vi "CSM with INI Config.vi"(5 "Init State(\"Macro: Initialize\")":string="Macro: Initialize", 7 "Name(\"\" to use uuid)":string="CSM-Module") -> ()   [LabVIEW 2017]
uses:
  269ea9ca-c704-454f-89fe-23bfb434a412.vi
  2c2747d1-7136-4018-a18b-7ed7b9b9eea8.vi
  <userlib>/_NEVSTOP/Communicable State Machine(CSM)/AdvanceAPI/CSM - Revert Arguments-Safe String.vi
  <userlib>/_NEVSTOP/Communicable State Machine(CSM)/AdvanceAPI/CSM - Make String Arguments Safe.vi
  <userlib>/_NEVSTOP/Communicable State Machine(CSM)/AdvanceAPI/CSM - Break Down Multiple States String.vi
  <userlib>/_NEVSTOP/Communicable State Machine(CSM)/AdvanceAPI/CSM - Compact Multiple States.vi
  269ea9ca-c704-454f-89fe-23bfb434a412.vi/b09b9099-6be0-413b-8afc-4908471460c3.vi
  2c2747d1-7136-4018-a18b-7ed7b9b9eea8.vi/99de0c97-112a-4c86-9094-c187659127e1.vi
  <userlib>/_NEVSTOP/Communicable State Machine(CSM)/AdvanceAPI/CSM - Keywords.vi
  <userlib>/_NEVSTOP/Communicable State Machine(CSM)/_Shared/Trim Single-line Text.vi
  INI-Static-Variable-Support/_Support/global-csm-ini-db-change-flag.vi
  <vilib>/Utility/Data Type/Get Type Information.vi
  <userlib>/_NEVSTOP/Communicable State Machine(CSM)/addons/API-String-Arugments-Support/_Support/Data To SingleElementsArray_csm.vi
  INI-Static-Variable-Support/_Support/Parse Used Session and Name.vi
  <userlib>/_NEVSTOP/Communicable State Machine(CSM)/addons/API-String-Arugments-Support/_Support/Data To API String Arguments.vi
  INI-Static-Variable-Support/_Support/INI-FGV(lvlibp).vi
  INI-Static-Variable-Support/_Support/Populate String with INI Variable.vi
  <userlib>/_NEVSTOP/Communicable State Machine(CSM)/addons/API-String-Arugments-Support/_Support/Convert API String Arguments to Data(variant).vi
  <userlib>/_NEVSTOP/Communicable State Machine(CSM)/addons/API-String-Arugments-Support/_Support/SingleElementsArray To Data_csm.vi
  <userlib>/_NEVSTOP/Communicable State Machine(CSM)/Communicable State Machine.lvlib
  INI-Static-Variable-Support/INI-Static-Variable-Support.lvlib
panel:
  in  "string":string
  out "State History":string
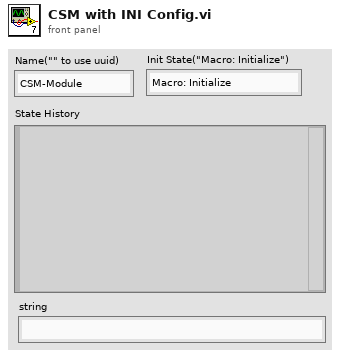
[diagram p1: front panel]
types:
  T1 = enum32{"Invalid", "Standard", "Closed", "Hidden", "Minimized", "Maximized"}
  T2 = enum32{"invalid app kind", "Development System", "Run Time System", "Student Edition", "Embedded LabVIEW", "Evaluation", "Custom"}
  T3 = typedef "Communicable State Machine.lvlib/_CSM_Response Source Message.ctl" = cluster{"‘State":string, "’Arguments":string, "’Error":errorcluster}
  T4 = cluster{"Core":cluster{"Current VI Reference":refnum<vi>, "Close Panel on Exit?":bool}, "Address":cluster{"IP":string, "Port":i16}, "Cert":cluster{"User":string, "Password":string}, "xxx":string}
  T5 = cluster{"Current VI Reference":refnum<vi>, "Close Panel on Exit?":bool}
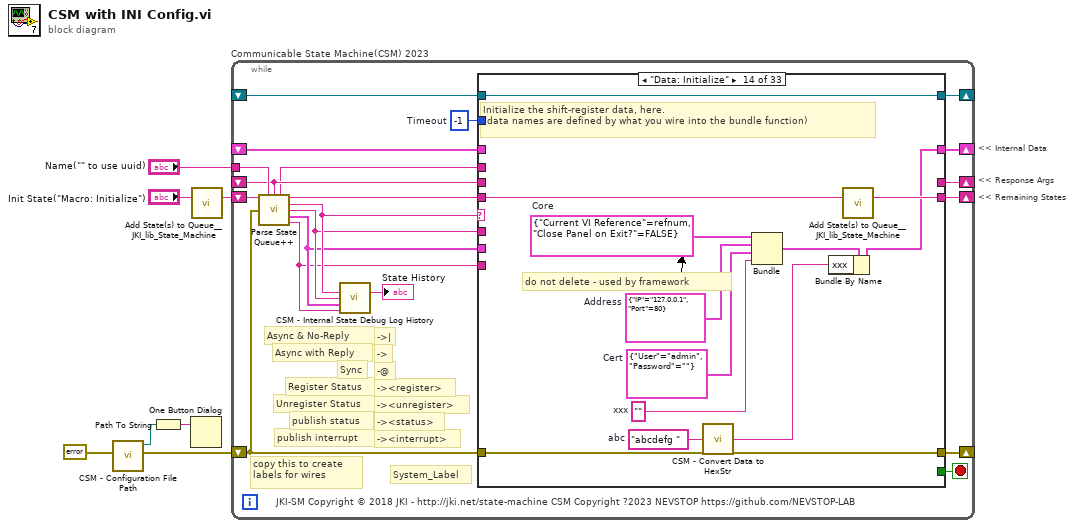
[diagram p0: block diagram]
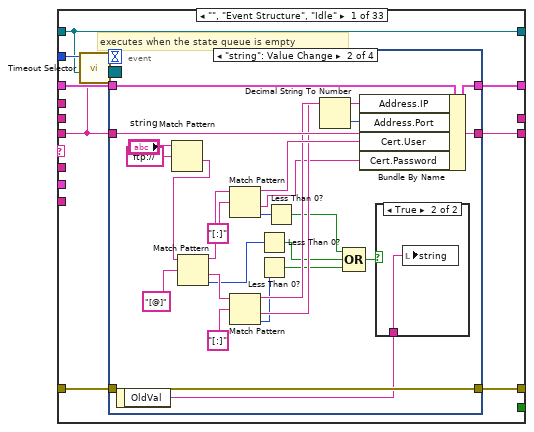
[diagram p2: hidden frame]
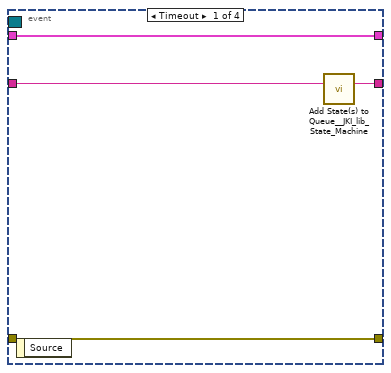
[diagram p3: hidden frame]
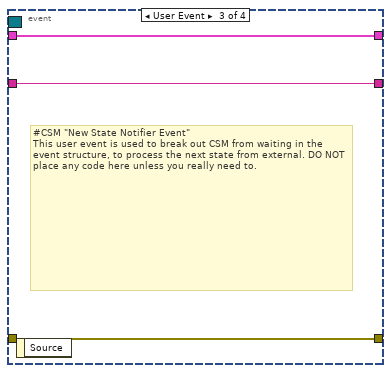
[diagram p5: hidden frame]
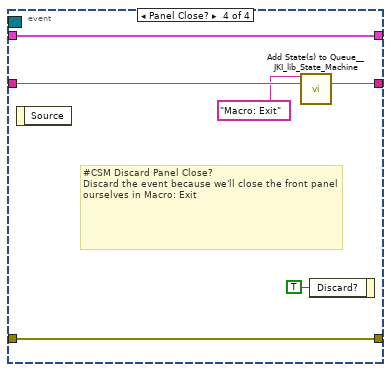
[diagram p6: hidden frame]
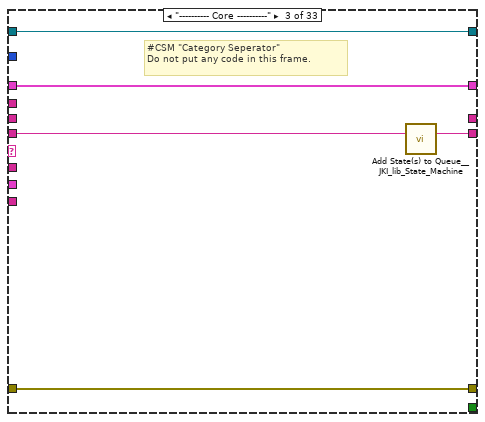
[diagram p8: hidden frame]
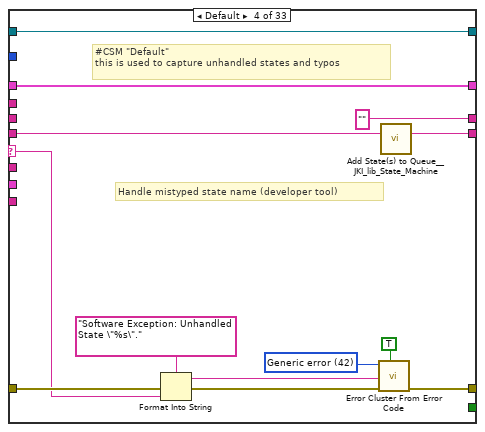
[diagram p9: hidden frame]
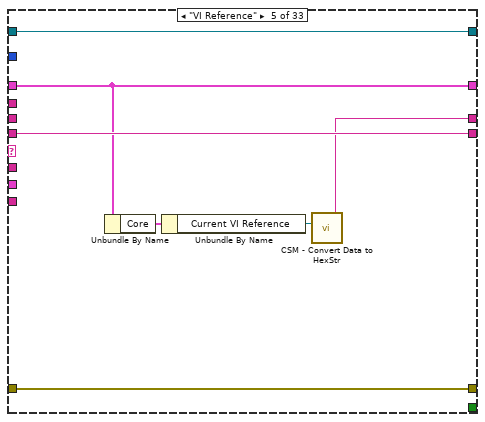
[diagram p10: hidden frame]
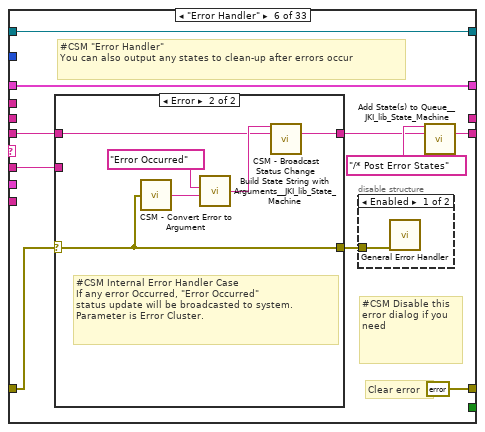
[diagram p11: hidden frame]
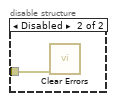
[diagram p12: hidden frame]
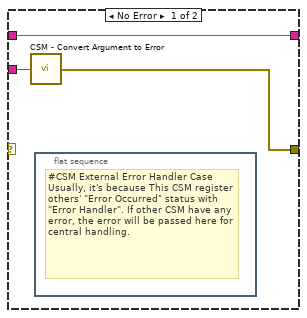
[diagram p13: hidden frame]
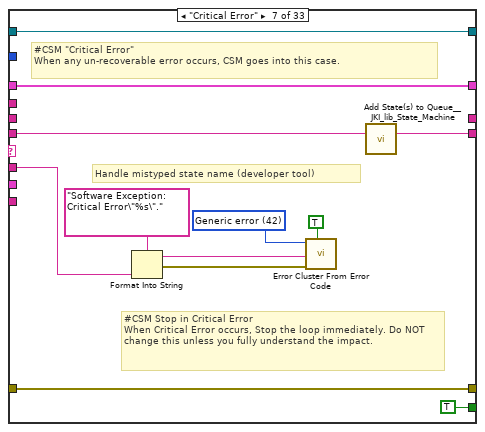
[diagram p14: hidden frame]
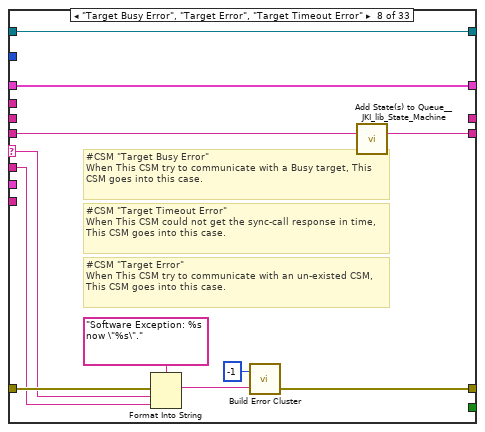
[diagram p15: hidden frame]
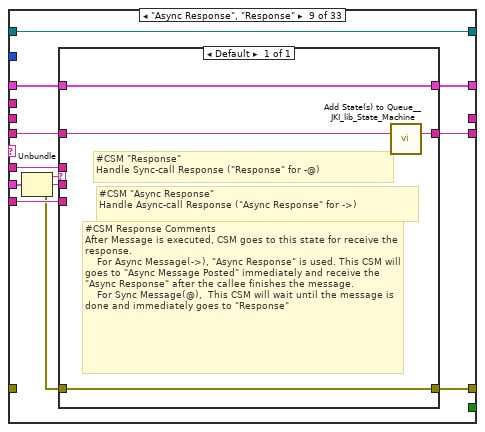
[diagram p16: hidden frame]
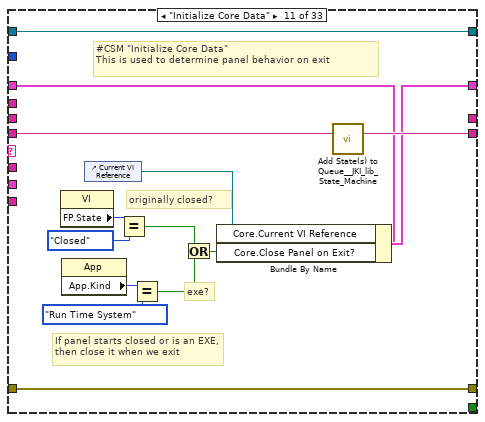
[diagram p18: hidden frame]
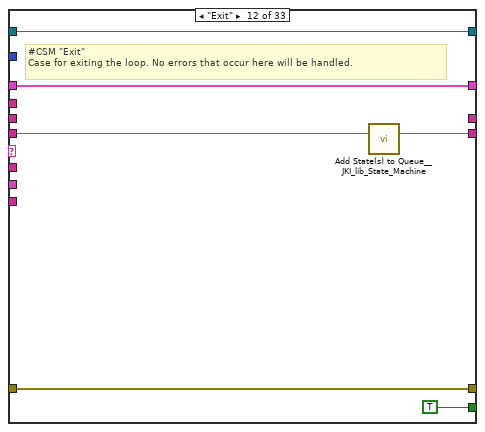
[diagram p19: hidden frame]
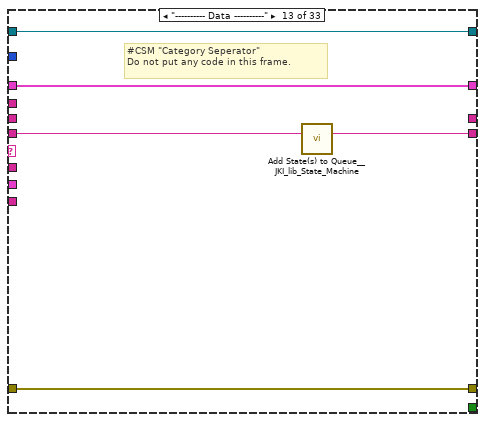
[diagram p20: hidden frame]
diagram:
  # "<< Internal Data"
  # "<< Response Args"
  # "<< Remaining States"
  n1 = call "CSM - Configuration File Path.vi"("error in (no error)"=errorcluster {"status"=FALSE, "code"=0, "source"=""} ("error out")) -> ("error out"=w3:errorcluster, "Default Config File Path"=w1:path)  [unwired: 6 in, 1 out]
  n2 = Path To String(path=w1) -> (string=w2:string)
  n3 = One Button Dialog(message=w2) -> ()  [unwired: 1 in, 1 out]
  n4 = call <vilib>:"Add State(s) to Queue__JKI_lib_State_Machine.vi"("State(s) in (\"\")"="Init State(\"Macro: Initialize\")") -> ("States Out"=w5:string)  [unwired: 14 in]
  n5 = while "Communicable State Machine(CSM) 2023" {
    shift-right: [w22] -> _
    shift-left: _ -> [w21]
    shift-right: [w25] -> _
    shift-left: w3 -> [w19]
    shift-right: [w24] -> _
    shift-left: w5 -> [w26]
    tunnel: "Name(\"\" to use uuid)" -> [w15]
    shift-right: [w18] -> _
    shift-left: _ -> [w10]
    shift-right: [w17] -> _
    shift-left: _ -> [w16]
    stop <- w23 stop-if-true
    w20 = -1  # Timeout
    # "-><interrupt>"
    # "-><status>"
    # "-><unregister>"
    # "-><register>"
    # "-@"
    # "->"
    # "->|"
    # "publish interrupt"
    # "publish status"
    # "Unregister Status"
    # "Register Status"
    # "Sync"
    # "Async with Reply"
    # "Async & No-Reply"
    # "copy this to create labels for wires"
    # "System_Label"
    # "JKI-SM Copyright © 2018 JKI - http://jki.net/state-machine CSM Copyright ?2023 NEVSTOP https://github.com/NEVSTOP-LAB"
    n6 = call <userlib>:"Parse State Queue++.vi"("State Queue"=w26, "Name (\"\" to Use UUID)"=w15, "Response Arguments"=w10, "Previous Error"=w19) -> ("Name Used"=w9:string, "Remaining States"=w27:string, "Current State"=w14:string, "Arguments"=w13:string, ">> Response Source Message >>"=w12:T3, ">> Source CSM >>"=w11:string)  [unwired: 6 in]
    n7 = call <userlib>:"CSM - Internal State Debug Log History.vi"("State"=w14, "Arguments (\"\")"=w13, ">> Response Source Message >>"=w12, "Source (\"\")"=w11) -> ("Debug Log"=→"State History":string)  [unwired: 11 in]
    n8 = case shown="\"Data: Initialize\"" w14 {
      selector: w14 -> [_ _ _ w87 _ _ _ w141 _ _ _ _ _ _ _ _ _ _ _ _ _ _ _ _ _ _ _ _ _ _ _ _ _]
      tunnel: w27 -> [w28 w78 w84 w91 w103 w109 w135 w143 w154 w167 w182 w188 w193 w205 w210 w217 w224 w229 w236 w240 w246 w257 w264 w280 w350 w356 w368 w371 w376 w382 w390 w396 w402]
      tunnel: w13 -> [_ _ _ _ _ w108 w128 w142 w153 _ _ _ _ _ _ _ _ _ _ _ _ _ w259 w274 _ _ _ _ _ w379 _ _ _]
      tunnel: w21 -> [w35 w77 w81 w89 w102 w113 w136 w145 w156 w166 w175 w186 w190 _ w208 w212 w219 w226 w235 w239 w243 w253 w262 w276 w347 w353 w365 w370 w375 w381 w387 w393 w399]
      tunnel: [w34 w79 w82 w93 w104 errorcluster {"status"=FALSE, "code"=0, "source"=""} ("error out") w137 w139 w159 w168 w179 w185 w191 w202 w211 w215 w220 w227 w230 w238 w244 w255 w260 w277 w348 w354 w366 w372 w377 w383 w388 w394 w400] -> w25
      tunnel: w19 -> [w33 w79 w82 w92 w104 w110 w137 w147 _ w168 w179 w185 w191 w202 w211 _ w221 w227 _ w241 w244 w255 w261 w278 w348 w354 w366 w372 w377 w383 w388 w394 w400]
      tunnel: [w36 w78 w83 w90 w103 w105 w134 w146 w155 w167 w181 w187 w192 w204 w210 w217 w223 w228 w236 w240 w245 w256 w263 w279 w349 w355 w367 w371 w376 w382 w389 w395 w401] -> w24
      tunnel: [_ _ _ _ _ _ TRUE _ _ _ _ TRUE _ _ _ _ _ _ _ _ _ _ _ _ _ _ _ _ _ _ _ _ _] -> w23
      tunnel: [w32 w77 w81 w89 w102 w113 w136 w145 w157 w166 w180 w186 w190 w195 w207 w213 w219 w226 w235 w239 w243 w253 w262 w276 w347 w353 w365 w370 w375 w381 w387 w393 w399] -> w22
      tunnel: w20 -> [w31 _ _ _ _ _ _ _ _ _ _ _ _ _ _ _ _ _ _ _ _ _ _ _ _ _ _ _ _ _ _ _ _]
      tunnel: w11 -> [_ _ _ _ _ _ _ _ w151 _ _ _ _ _ _ _ _ _ _ _ _ _ _ _ _ _ _ _ _ _ _ _ _]
      tunnel: w12 -> [_ _ _ _ _ _ _ _ w158 _ _ _ _ _ _ _ _ _ _ _ _ _ _ _ _ _ _ _ _ _ _ _ _]
      tunnel: [_ _ _ "" w98 _ _ _ _ _ _ _ _ _ _ _ _ _ _ _ _ _ _ _ _ _ _ _ "API1 Response" w378 _ "DoA Finished" "DoB Finished"] -> w18
      tunnel: [w30 w76 w80 w85 w101 w112 w126 w144 w160 w165 w169 w183 w189 w200 w209 w216 w218 w225 w234 w237 w242 w254 w258 w273 w346 w351 w358 w369 w374 w380 w386 w392 w398] -> w17
      tunnel: w16 -> [w30 w76 w80 w85 w101 w112 w126 w144 w160 w165 w169 w183 w189 w200 w209 w216 w218 w225 _ w237 w242 w254 w258 w273 w346 w351 w358 w369 w374 w380 w386 w392 w398]
      tunnel: w10 -> [_ _ _ _ _ _ _ _ _ _ _ _ _ _ _ _ _ _ _ _ _ _ _ _ _ _ _ _ _ _ _ _ _]
      tunnel: w9 -> [_ _ _ _ _ _ _ _ _ _ _ _ _ _ w206 w214 _ _ w233 _ _ _ _ _ _ _ _ _ _ _ _ _ _]
      frame "", "Event Structure", "Idle" {
        # "executes when the state queue is empty"
        n9 = call <userlib>:"Timeout Selector.vi"("Remaining States"=w28, "Timeout Expected"=w31) -> ("Timeout"=w29:i32)  [unwired: 5 in]
        n10 = event shown="[1] \"string\": Value Change" {
          selector: w30 -> [_ _ _ _]
          dyn-events: _ -> [_ _ _ _]
          timeout: w29 -> [_ _ _ _]
          tunnel: w28 -> [w40 w65 w68 w75]
          tunnel: [w39 w65 w68 w74] -> w36
          tunnel: w35 -> [w37 w63 w69 w72]
          tunnel: [w38 w64 w67 w73] -> w34
          tunnel: w33 -> [w38 w64 w67 w73]
          tunnel: [w37 w61 w69 w72] -> w32
          event Timeout {
            n11 = event-data() -> ()  [unwired: 1 in, 1 out]
            n12 = call <vilib>:"Add State(s) to Queue__JKI_lib_State_Machine.vi"("State(s) in (\"\")"=w40) -> ("States Out"=w39:string)  [unwired: 14 in]
          }
          event "string": Value Change {
            n13 = event-data() -> ("OldVal"=w62:string)  [unwired: 1 in]
            n14 = Match Pattern(string="string", regular expression="ftp://") -> (after substring=w42:string)  [unwired: 1 in, 3 out]
            n15 = Match Pattern(string=w42, regular expression="[@]") -> (before substring=w58:string, after substring=w56:string, offset past match=w51:i32)  [unwired: 1 in, 1 out]
            n16 = Match Pattern(string=w58, regular expression="[:]") -> (before substring=w55:string, after substring=w41:string, offset past match=w50:i32)  [unwired: 1 in, 1 out]
            n17 = Match Pattern(string=w56, regular expression="[:]") -> (before substring=w54:string, after substring=w53:string, offset past match=w49:i32)  [unwired: 1 in, 1 out]
            n18 = Less Than 0?(x=w51) -> (x < 0?=w46:bool)
            n19 = Less Than 0?(x=w49) -> (x < 0?=w45:bool)
            n20 = Less Than 0?(x=w50) -> (x < 0?=w47:bool)
            n21 = Decimal String To Number(string=w53) -> (number=w52:i32)  [unwired: 2 in, 1 out]
            n22 = Compound Arithmetic op=OR(w47, w46, w45) -> (w48:bool)
            n23 = Bundle By Name(cluster=w63, "Address.IP"=w54, "Address.Port"=w52, "Cert.User"=w55, "Cert.Password"=w41) -> (w61:T4)
            n24 = case shown="True" w48 {
              tunnel: w62 -> [_ w66]
              frame False {
              }
              frame True {
                n25 = local write "string"(w66) -> ()
              }
            }
          }
          event User Event {
            # "#CSM \"New State Notifier Event\"\nThis user event is used to break out CSM from waiting in the event structure, to process the next state from external. DO NOT place any code here unless you really need to."
            n26 = event-data() -> ()  [unwired: 1 in, 1 out]
          }
          event Panel Close? {
            # "#CSM Discard Panel Close?\nDiscard the event because we'll close the front panel ourselves in Macro: Exit"
            n27 = event-data() -> ()  [unwired: 1 in, 1 out]
            n28 = call <vilib>:"Add State(s) to Queue__JKI_lib_State_Machine.vi"("State(s) in Front (\"\")"="Macro: Exit", "State(s) in (\"\")"=w75) -> ("States Out"=w74:string)  [unwired: 13 in]
            n29 = event-data("Discard?"=TRUE) -> ()  [unwired: 1 in, 1 out]
          }
        }
      }
      frame "CSM Documentation" {
        # "#CSM README FIRST\n\nCSM is a LabVIEW application framework that builds upon JKI State Machine (JKISM). It follows the pattern of JKISM and extends the keywords to describe message communication between CSM modules, including concepts such as Sync-Message, Async-Message, Subscription/Unsubscription of status - essential elements for creating reusable code modules. For more information, please visit the CSM wiki: https://github.com/NEVSTOP-LAB/JKI-State-Machine-Plus-Plus/wiki\n\nFor instructions on JKI State Machine, visit: http://jki.net/state-machine/\nFor information about CSM, visit: https://github.com/NEVSTOP-LAB"
        # "#CSM \"Documentation\"\nCase for holding CSM Documenation"
      }
      frame "---------- Core ----------" {
        # "#CSM \"Category Seperator\"\nDo not put any code in this frame."
        n30 = call <vilib>:"Add State(s) to Queue__JKI_lib_State_Machine.vi"("State(s) in (\"\")"=w84) -> ("States Out"=w83:string)  [unwired: 14 in]
      }
      frame Default {
        w96 = 42 items=["No error", "Argument error", "Memory is full", "Out of zone", "End of file", "File already open", "Generic file I/O error", "File not found", "File permission error", "Disk is full", "Duplicate path", "Too many files open", "System feature not enabled", "Resource file not found", "Cannot add resource", "Resource not found", "Image not found", "Image memory error", "Pen does not exist", "Config type invalid", "Config token not found", "Config parse error", "Config memory error", "Bad external code format", "Bad external code offset", "External code not present", "Null window", "Destroy window error", "Null menu", "Print aborted", "Bad print record", "Print driver error", "Windows error during printing", "Memory error during printing", "Print dialog error", "Generic print error", "Invalid device refnum", "Device not found", "Device parameter error", "Device unit error", "Cannot open device", "Device call aborted", "Generic error", "Cancelled by user", "Object ID too low", "Object ID too high", "Object not in heap", "Unknown heap", "Unknown object (invalid DefProc)", "Unknown object (DefProc not in table)", "Message out of range", "Invalid (null) method", "Unknown message", "Manager call not supported", "Bad address", "Network operation in progress", "Network operation timed out", "Connection is busy", "Network attribute not supported", "Network error", "Address in use", "System out of memory", "Connection aborted", "Connection refused", "Not connected", "Already connected", "Connection closed", "Initialization error (interapplication manager)", "Bad occurrence", "Wait on unbound occurrence handler", "Occurrence queue overflow", "Datalog type conflict", "Unused", "Unrecognized type (interapplication manager)", "Memory corrupt", "Failed to make temporary DLL", "Old CIN version", "Drag socket not found", "Failed to load drop-object", "Failed to register OLE object", "Failed to release OLE object", "Format specifier type mismatch", "Unknown format specifier", "Too few format specifiers", "Too many format specifiers", "Scan failed", "Newer CIN version", "Error converting to variant", "Runtime menu error", "Password tampered", "Variant attribute not found", "Incompatible variant data type", "Event data is not available", "Event Store is not present", "Occurrence is not found", "Event Queue is not created", "Event info is not available", "Refnum passed is NULL", "Error retrieving Class GUID", "Error retrieving CoClass GUID", "Error retrieving TypeLib GUID.", "Bad built application magic bytes.", "Specific driver is different from the specific driver associated with the Logical Name.", "There is no session opened to the class driver.", "Max Error", "MAX - Error with config objects", "MAX - Error loading configuration", "MAX - Group not supported"]
        # "#CSM \"Default\"\nthis is used to capture unhandled states and typos"
        # "Handle mistyped state name (developer tool)"
        n31 = Format Into String(format string="Software Exception: Unhandled State \"%s\"." ("message"), error in=w92, w87) -> (resulting string=w95:string, error out=w94:errorcluster)  [unwired: 1 in]
        n32 = call <vilib>:"Error Cluster From Error Code.vi"("show call chain? (False)"=TRUE, "error in (no error)"=w94, "error message (\"\")"=w95, "error code (0)"=w96) -> ("error out"=w93:errorcluster)  [unwired: 5 in]
        n33 = call <vilib>:"Add State(s) to Queue__JKI_lib_State_Machine.vi"("State(s) in (\"\")"=w91) -> ("States Out"=w90:string)  [unwired: 14 in]
      }
      frame "VI Reference" {
        n34 = Unbundle By Name(w102) -> ("Core"=w100:T5)
        n35 = Unbundle By Name(w100) -> ("Current VI Reference"=w99:refnum<vi>)
        n36 = call <userlib>:"CSM - Convert Data to HexStr.vi"("Variant"=w99) -> ("HEX String (0-9,A-F)"=w98:string)  [unwired: 8 in]
      }
      frame "Error Handler" {
        # "#CSM Disable this error dialog if you need"
        # "#CSM \"Error Handler\"\nYou can also output any states to clean-up after errors occur"
        # "Clear error"
        n37 = case shown="Error" w110 {
          selector: w110 -> [_ w120]
          tunnel: [w119 w122] -> w106
          tunnel: w109 -> [w119 w121]
          tunnel: w108 -> [w118 _]
          tunnel: [w117 w120] -> w111
          frame No Error {
            n38 = call <userlib>:"CSM - Convert Argument to Error.vi"("Argument"=w118) -> ("Error"=w117:errorcluster)  [unwired: 4 in]
            n39 = flat-sequence {
              frame #0 {
                # "#CSM External Error Handler Case\nUsually, it's because This CSM register others' \"Error Occurred\" status with \"Error Handler\". If other CSM have any error, the error will be passed here for central handling."
              }
            }
          }
          frame Error {
            # "#CSM Internal Error Handler Case \nIf any error Occurred, \"Error Occurred\" \nstatus update will be broadcasted to system.\nParameter is Error Cluster."
            n40 = call <userlib>:"CSM - Convert Error to Argument.vi"("Error"=w120) -> ("Argument"=w124:string)  [unwired: 4 in]
            n41 = call <vilib>:"Build State String with Arguments__JKI_lib_State_Machine.vi"("Arguments (\"\")"=w124, "State"="Error Occurred" ("Status with Arguments")) -> ("State with Arguments"=w123:string)  [unwired: 4 in]
            n42 = call <userlib>:"CSM - Broadcast Status Change.vi"("Status With Arguments"=w123, "State Queue"=w121) -> ("Remaining States"=w122:string)  [unwired: 13 in]
          }
        }
        n43 = disable-structure shown="Enabled" {
          disable-tunnel: w111 -> [w115 w116]
          frame Enabled {
            n44 = call <vilib>:"General Error Handler.vi"("error in (no error)"=w115) -> ()  [unwired: 10 in, 5 out]
          }
          frame Disabled {
            n45 = call <vilib>:"Clear Errors.vi"("error in (no error)"=w116) -> ()  [unwired: 5 in, 2 out]
          }
        }
        n46 = call <vilib>:"Add State(s) to Queue__JKI_lib_State_Machine.vi"("State(s) in Front (\"\")"="/* Post Error States", "State(s) in (\"\")"=w106) -> ("States Out"=w105:string)  [unwired: 13 in]
      }
      frame "Critical Error" {
        w132 = 42 items=["No error", "Argument error", "Memory is full", "Out of zone", "End of file", "File already open", "Generic file I/O error", "File not found", "File permission error", "Disk is full", "Duplicate path", "Too many files open", "System feature not enabled", "Resource file not found", "Cannot add resource", "Resource not found", "Image not found", "Image memory error", "Pen does not exist", "Config type invalid", "Config token not found", "Config parse error", "Config memory error", "Bad external code format", "Bad external code offset", "External code not present", "Null window", "Destroy window error", "Null menu", "Print aborted", "Bad print record", "Print driver error", "Windows error during printing", "Memory error during printing", "Print dialog error", "Generic print error", "Invalid device refnum", "Device not found", "Device parameter error", "Device unit error", "Cannot open device", "Device call aborted", "Generic error", "Cancelled by user", "Object ID too low", "Object ID too high", "Object not in heap", "Unknown heap", "Unknown object (invalid DefProc)", "Unknown object (DefProc not in table)", "Message out of range", "Invalid (null) method", "Unknown message", "Manager call not supported", "Bad address", "Network operation in progress", "Network operation timed out", "Connection is busy", "Network attribute not supported", "Network error", "Address in use", "System out of memory", "Connection aborted", "Connection refused", "Not connected", "Already connected", "Connection closed", "Initialization error (interapplication manager)", "Bad occurrence", "Wait on unbound occurrence handler", "Occurrence queue overflow", "Datalog type conflict", "Unused", "Unrecognized type (interapplication manager)", "Memory corrupt", "Failed to make temporary DLL", "Old CIN version", "Drag socket not found", "Failed to load drop-object", "Failed to register OLE object", "Failed to release OLE object", "Format specifier type mismatch", "Unknown format specifier", "Too few format specifiers", "Too many format specifiers", "Scan failed", "Newer CIN version", "Error converting to variant", "Runtime menu error", "Password tampered", "Variant attribute not found", "Incompatible variant data type", "Event data is not available", "Event Store is not present", "Occurrence is not found", "Event Queue is not created", "Event info is not available", "Refnum passed is NULL", "Error retrieving Class GUID", "Error retrieving CoClass GUID", "Error retrieving TypeLib GUID.", "Bad built application magic bytes.", "Specific driver is different from the specific driver associated with the Logical Name.", "There is no session opened to the class driver.", "Max Error", "MAX - Error with config objects", "MAX - Error loading configuration", "MAX - Group not supported"]
        # "#CSM Stop in Critical Error\nWhen Critical Error occurs, Stop the loop immediately. Do NOT change this unless you fully understand the impact."
        # "#CSM \"Critical Error\"\nWhen any un-recoverable error occurs, CSM goes into this case."
        # "Handle mistyped state name (developer tool)"
        n47 = Format Into String(format string="Software Exception: Critical Error\"%s\"." ("message"), w128) -> (resulting string=w131:string, error out=w130:errorcluster)  [unwired: 2 in]
        n48 = call <vilib>:"Error Cluster From Error Code.vi"("show call chain? (False)"=TRUE, "error in (no error)"=w130, "error message (\"\")"=w131, "error code (0)"=w132) -> ()  [unwired: 5 in, 1 out]
        n49 = call <vilib>:"Add State(s) to Queue__JKI_lib_State_Machine.vi"("State(s) in (\"\")"=w135) -> ("States Out"=w134:string)  [unwired: 14 in]
      }
      frame "Target Busy Error", "Target Error", "Target Timeout Error" {
        # "#CSM \"Target Error\"\nWhen This CSM try to communicate with an un-existed CSM, This CSM goes into this case."
        # "#CSM \"Target Timeout Error\"\nWhen This CSM could not get the sync-call response in time, This CSM goes into this case."
        # "#CSM \"Target Busy Error\"\nWhen This CSM try to communicate with a Busy target, This CSM goes into this case."
        n50 = Format Into String(format string="Software Exception: %s now \"%s\"." ("message"), error in=w147, w141, w142) -> (resulting string=w140:string)  [unwired: 1 in, 1 out]
        n51 = call <userlib>:"Build Error Cluster.vi"("String to Prepend to Source (\"\")"=w140, "Code"=-1 ("code")) -> ("error out"=w139:errorcluster)
        n52 = call <vilib>:"Add State(s) to Queue__JKI_lib_State_Machine.vi"("State(s) in (\"\")"=w143) -> ("States Out"=w146:string)  [unwired: 14 in]
      }
      frame "Async Response", "Response" {
        n53 = Unbundle(w158) -> ("‘State"=w152:string, "’Arguments"=w150:string, "’Error"=w149:errorcluster)
        n54 = case shown="Default" w152 {
          tunnel: [w164] -> w159
          tunnel: w149 -> [w164]
          tunnel: [w163] -> w157
          tunnel: w156 -> [w163]
          tunnel: [w161] -> w155
          tunnel: w154 -> [w162]
          tunnel: w153 -> [_]
          tunnel: w151 -> [_]
          tunnel: w150 -> [_]
          frame Default {
            # "#CSM Response Comments\nAfter Message is executed, CSM goes to this state for receive the response.\n    For Async Message(->), \"Async Response\" is used. This CSM will goes to \"Async Message Posted\" immediately and receive the \"Async Response\" after the callee finishes the message.\n    For Sync Message(@),  This CSM will wait until the message is done and immediately goes to \"Response\""
            # "#CSM \"Async Response\"\nHandle Async-call Response (\"Async Response\" for ->)"
            # "#CSM \"Response\"\nHandle Sync-call Response (\"Response\" for -@)"
            n55 = call <vilib>:"Add State(s) to Queue__JKI_lib_State_Machine.vi"("State(s) in (\"\")"=w162) -> ("States Out"=w161:string)  [unwired: 14 in]
          }
        }
      }
      frame "Async Message Posted" {
        # "#CSM \"Async Message Posted\"\nAfter Async Message is posted (-> or ->| ), CSM goes to this state for post-action.\nYou can use Argument - State to tell which Async Message is called."
      }
      frame "Initialize Core Data" {
        # "#CSM \"Initialize Core Data\"\nThis is used to determine panel behavior on exit"
        # "originally closed?"
        # "exe?"
        # "If panel starts closed or is an EXE, then close it when we exit"
        n56 = property class="VI"() -> ("FP.State"=w172:T1)  [unwired: 2 in, 2 out]
        n57 = property class="App"() -> ("App.Kind"=w178:T2)  [unwired: 2 in, 2 out]
        n58 = control-ref of="Current VI Reference"() -> (w173:refnum<vi>)
        n59 = Equal?(x=w172, y=T1."Closed" ("Front Panel Window:State")) -> (x = y?=w170:bool)
        n60 = Equal?(x=w178, y=T2."Run Time System" ("Application:Kind")) -> (x = y?=w176:bool)
        n61 = Or(x=w170, y=w176) -> (x .or. y?=w174:bool)
        n62 = Bundle By Name(cluster=w175, "Core.Current VI Reference"=w173, "Core.Close Panel on Exit?"=w174) -> (w180:T4)
        n63 = call <vilib>:"Add State(s) to Queue__JKI_lib_State_Machine.vi"("State(s) in (\"\")"=w182) -> ("States Out"=w181:string)  [unwired: 14 in]
      }
      frame "Exit" {
        # "#CSM \"Exit\"\nCase for exiting the loop. No errors that occur here will be handled."
        n64 = call <vilib>:"Add State(s) to Queue__JKI_lib_State_Machine.vi"("State(s) in (\"\")"=w188) -> ("States Out"=w187:string)  [unwired: 14 in]
      }
      frame "---------- Data ----------" {
        # "#CSM \"Category Seperator\"\nDo not put any code in this frame."
        n65 = call <vilib>:"Add State(s) to Queue__JKI_lib_State_Machine.vi"("State(s) in (\"\")"=w193) -> ("States Out"=w192:string)  [unwired: 14 in]
      }
      frame "Data: Initialize" {
        w196 = "abcdefg "  # abc
        w197 = ""  # xxx
        w198 = cluster{"User":string, "Password":string} {"User"="admin", "Password"=""}  # Cert
        w199 = cluster{"IP":string, "Port":i16} {"IP"="127.0.0.1", "Port"=80}  # Address
        w201 = T5 {"Current VI Reference"=refnum, "Close Panel on Exit?"=FALSE}  # Core
        # "do not delete - used by framework"
        # "Initialize the shift-register data, here.\n(data names are defined by what you wire into the bundle function)"
        n66 = call <userlib>:"CSM - Convert Data to HexStr.vi"("Variant"=w196) -> ("HEX String (0-9,A-F)"=w194:string)  [unwired: 8 in]
        n67 = Bundle("Core"=w201, "Address"=w199, "Cert"=w198, "xxx"=w197) -> (w203:T4)  [unwired: 1 in]
        n68 = Bundle By Name(cluster=w203, "xxx"=w194) -> (w195:T4)
        n69 = call <vilib>:"Add State(s) to Queue__JKI_lib_State_Machine.vi"("State(s) in (\"\")"=w205) -> ("States Out"=w204:string)  [unwired: 14 in]
      }
      frame "Data: Load From INI" {
        n70 = call "CSM - Read Configuration Variable.vim"("Section Name(\"\" as Default)"=w206, "config prototype(Cluster Prefered)"=w208) -> ("config out"=w207:T4)  [unwired: 6 in, 1 out]
      }
      frame "Data: Save to INI" {
        n71 = call "CSM - Write Configuration Variable.vim"("Section Name(\"\" as Default)"=w214, "Variant"=w212) -> ("error out"=w215:errorcluster, "Variant (dup)"=w213:T4)  [unwired: 6 in]
      }
      frame "Data: Cleanup" {
        # "Cleanup any data and references, here.\n(this is called automatically, by the Macro: Exit)"
        n72 = Unbundle By Name(w219) -> ("Core.Current VI Reference"=w222:refnum<vi>)
        n73 = Close Reference(reference=w222, error in (no error)=w221) -> (error out=w220:errorcluster)
        n74 = call <vilib>:"Add State(s) to Queue__JKI_lib_State_Machine.vi"("State(s) in (\"\")"=w224) -> ("States Out"=w223:string)  [unwired: 14 in]
      }
      frame "---------- Events ----------" {
        # "#CSM \"Category Seperator\"\nDo not put any code in this frame."
        n75 = call <vilib>:"Add State(s) to Queue__JKI_lib_State_Machine.vi"("State(s) in (\"\")"=w229) -> ("States Out"=w228:string)  [unwired: 14 in]
      }
      frame "Events: Register" {
        # "#CSM \"Events: Register\"\nRegister user event. New Message Event is registered to break CSM waiting in event structure by default."
        # "#CSM Register New Message Event\nRegister message event to break Waiting in Event structure."
        n76 = call <userlib>:"CSM - Get New State Notifier Event.vi"("Name (\"\" to Use UUID) In"=w233) -> ("error out"=w231:errorcluster, "New State Notifier Event"=w232:refnum<user-event>)  [unwired: 9 in]
        n77 = register-events(error in=w231, w232) -> (reference out=w234:refnum<event-registration>, error out=w230:errorcluster)  [unwired: 1 in]
      }
      frame "Events: Unregister" {
        # "#CSM \"Events: Unregister\"\nUnregister user event."
        n78 = Unregister For Events(event registration refnum=w237, error in=w241) -> (error out=w238:errorcluster)
      }
      frame "---------- UI ----------" {
        # "#CSM \"Category Seperator\"\nDo not put any code in this frame."
        n79 = call <vilib>:"Add State(s) to Queue__JKI_lib_State_Machine.vi"("State(s) in (\"\")"=w246) -> ("States Out"=w245:string)  [unwired: 14 in]
      }
      frame "UI: Initialize" {
        # "#CSM \"UI: Initialize\"\nInitialize the User Interface, here.\n(this is called automatically, by the Macro: Init)"
        n80 = Unbundle By Name(w253) -> ("Address.IP"=w249:string, "Address.Port"=w248:i16, "Cert.User"=w251:string, "Cert.Password"=w250:string)
        n81 = Format Into String(format string="ftp://%s:%s@%s:%d", w251, w250, w249, w248) -> (resulting string=w247:string)  [unwired: 2 in, 1 out]
        n82 = call <vilib>:"Add State(s) to Queue__JKI_lib_State_Machine.vi"("State(s) in (\"\")"=w257) -> ("States Out"=w256:string)  [unwired: 14 in]
        n83 = local write "string"(w247) -> ()
      }
      frame "UI: Cursor Set" {
        # "#CSM \"UI: Cursor Set\"\nSet and Unset Cursor Busy.\n(Usage: \"UI: Cursor Set >> Busy|Idle\")"
        # "Argument"
        n84 = disable-structure shown="Default" {
          disable-tunnel: w261 -> [w267 w272]
          disable-tunnel: [w266 w272] -> w260
          disable-tunnel: w259 -> [w265 _]
          frame condition #0 (active) {
            n85 = case shown="\"Idle\", Default" w265 {
              tunnel: w267 -> [w269 w271]
              tunnel: [w268 w270] -> w266
              frame "Idle", Default {
                n86 = call <vilib>:"Unset Busy.vi"("error in (no error)"=w269) -> ("error out"=w268:errorcluster)  [unwired: 10 in]
              }
              frame "Busy" {
                n87 = call <vilib>:"Set Busy.vi"("error in (no error)"=w271) -> ("error out"=w270:errorcluster)  [unwired: 9 in, 1 out]
              }
            }
          }
          frame condition #1 {
          }
        }
        n88 = call <vilib>:"Add State(s) to Queue__JKI_lib_State_Machine.vi"("State(s) in (\"\")"=w264) -> ("States Out"=w263:string)  [unwired: 14 in]
      }
      frame "UI: Front Panel State" {
        # "#CSM \"UI: Front Panel State\"\nSet Front Panel Open or Closed\n(Usage: \"UI: Front Panel State >> Open|Close\")"
        # "Argument"
        n89 = Unbundle By Name(w276) -> ("Core.Current VI Reference"=w275:refnum<vi>)
        n90 = call <vilib>:"Add State(s) to Queue__JKI_lib_State_Machine.vi"("State(s) in (\"\")"=w280) -> ("States Out"=w279:string)  [unwired: 14 in]
        n91 = case shown="\"Close\", \"Closed\"" w274 {
          tunnel: w278 -> [w286 w301 w312 w325 w338]
          tunnel: [w288 w302 w314 w327 w340] -> w277
          tunnel: w275 -> [w287 w299 w313 w326 w339]
          frame "Open", "Standard", Default {
            w281 = T1."Standard" ("State")
            n92 = property class="VI"(reference=w287, error in=w286) -> (reference out=w284:refnum<vi>, error out=w285:errorcluster, "FP.State"=w283:T1)
            n93 = Not Equal?(x=w283, y=w281) -> (x != y?=w282:bool)
            n94 = case shown="True" w282 {
              tunnel: [w292 w294] -> w288
              tunnel: w285 -> [w291 w294]
              tunnel: w284 -> [w290 _]
              tunnel: w281 -> [w289 _]
              frame True {
                n95 = invoke class="VI" method="FP.Open"(reference=w290, error in=w291, "Activate"=TRUE, "State"=w289) -> (error out=w292:errorcluster)  [unwired: 1 in, 4 out]
              }
              frame False {
              }
            }
          }
          frame "Close", "Closed" {
            n96 = property class="VI"(reference=w299, error in=w301) -> (reference out=w298:refnum<vi>, error out=w300:errorcluster, "FP.State"=w296:T1)
            n97 = Not Equal?(x=w296, y=T1."Closed" ("Front Panel Window:State")) -> (x != y?=w295:bool)
            n98 = case shown="False" w295 {
              tunnel: [w303 w306] -> w302
              tunnel: w300 -> [w303 w305]
              tunnel: w298 -> [_ w304]
              frame False {
              }
              frame True {
                n99 = invoke class="VI" method="FP.Close"(reference=w304, error in=w305) -> (error out=w306:errorcluster)  [unwired: 1 in, 2 out]
              }
            }
          }
          frame "Hidden", "Hide" {
            w307 = T1."Hidden" ("State")
            n100 = property class="VI"(reference=w313, error in=w312) -> (reference out=w310:refnum<vi>, error out=w311:errorcluster, "FP.State"=w309:T1)
            n101 = Not Equal?(x=w309, y=w307) -> (x != y?=w308:bool)
            n102 = case shown="True" w308 {
              tunnel: [w318 w319] -> w314
              tunnel: w311 -> [w317 w319]
              tunnel: w310 -> [w316 _]
              tunnel: w307 -> [w315 _]
              frame True {
                n103 = invoke class="VI" method="FP.Open"(reference=w316, error in=w317, "State"=w315) -> (error out=w318:errorcluster)  [unwired: 2 in, 4 out]
              }
              frame False {
              }
            }
          }
          frame "Minimize", "Minimized" {
            w320 = T1."Minimized" ("State")
            n104 = property class="VI"(reference=w326, error in=w325) -> (reference out=w323:refnum<vi>, error out=w324:errorcluster, "FP.State"=w322:T1)
            n105 = Not Equal?(x=w322, y=w320) -> (x != y?=w321:bool)
            n106 = case shown="True" w321 {
              tunnel: [w331 w332] -> w327
              tunnel: w324 -> [w330 w332]
              tunnel: w323 -> [w329 _]
              tunnel: w320 -> [w328 _]
              frame True {
                n107 = invoke class="VI" method="FP.Open"(reference=w329, error in=w330, "State"=w328) -> (error out=w331:errorcluster)  [unwired: 2 in, 4 out]
              }
              frame False {
              }
            }
          }
          frame "Maximize", "Maximized" {
            w333 = T1."Maximized" ("State")
            n108 = property class="VI"(reference=w339, error in=w338) -> (reference out=w336:refnum<vi>, error out=w337:errorcluster, "FP.State"=w335:T1)
            n109 = Not Equal?(x=w335, y=w333) -> (x != y?=w334:bool)
            n110 = case shown="True" w334 {
              tunnel: [w344 w345] -> w340
              tunnel: w337 -> [w343 w345]
              tunnel: w336 -> [w342 _]
              tunnel: w333 -> [w341 _]
              frame True {
                n111 = invoke class="VI" method="FP.Open"(reference=w342, error in=w343, "State"=w341) -> (error out=w344:errorcluster)  [unwired: 2 in, 4 out]
              }
              frame False {
              }
            }
          }
        }
      }
      frame "---------- Macro ----------" {
        # "#CSM \"Category Seperator\"\nDo not put any code in this frame."
        n112 = call <vilib>:"Add State(s) to Queue__JKI_lib_State_Machine.vi"("State(s) in (\"\")"=w350) -> ("States Out"=w349:string)  [unwired: 14 in]
      }
      frame "Macro: Initialize" {
        w352 = "Data: Initialize\nData: Load From INI\nInitialize Core Data\nEvents: Register\nUI: Initialize\nUI: Front Panel State >> Open"  # Data: Initialize Data: Load From INI Initialize Core Data Events: Register UI: Initialize UI: Front Panel State >> Open
        # "#CSM \"Macro: Initialize\"\nInitialization Macro (This is called once, when the VI starts)"
        n113 = call <vilib>:"Add State(s) to Queue__JKI_lib_State_Machine.vi"("State(s) in Front (\"\")"=w352, "State(s) in (\"\")"=w356) -> ("States Out"=w355:string)  [unwired: 13 in]
      }
      frame "Macro: Exit" {
        # "#CSM \"Macro: Exit\"\nExit Macro (This is called once, when the VI exits)"
        n114 = Unbundle By Name(w365) -> ("Core.Close Panel on Exit?"=w364:bool)
        n115 = Select(t="UI: Front Panel State >> Close", s=w364, f="") -> (s? t:f=w361:string)
        n116 = call <vilib>:"Add State(s) to Queue__JKI_lib_State_Machine.vi"("State(s) in Front (\"\")"="Data: Save to INI\n//Exit Sub-Modules ", "State(s) in (\"\")"=w361, "State(s) at Back (\"\")"="Data: Cleanup\nEvents: Unregister\nExit") -> ("States Out"=w359:string)  [unwired: 12 in]
        n117 = call <vilib>:"Add State(s) to Queue__JKI_lib_State_Machine.vi"("State(s) in Front (\"\")"=w359, "State(s) in (\"\")"=w368) -> ("States Out"=w367:string)  [unwired: 13 in]
      }
      frame "---------- API ----------" {
        # "#CSM \"Category Seperator\"\nDo not put any code in this frame."
      }
      frame "API: API1" {
        # "#CSM API Example\nCopy/Rename this case for your own API"
        # "#CSM Response\nConnect this to return the response of your API"
        # "#CSM >> Source CSM >>\nIf you need to tell who triggered this state , use this string. If it's this case itself, this string is \"\"."
        # "#CSM >> Arguments >>\nDeal with the parameter if any"
      }
      frame "API: API2" {
        # "#CSM API Example\nCopy/Rename this case for your own API"
        # "unpack Hex String  to Variant\nif complex parameter is needed."
        n118 = call <userlib>:"CSM - Convert HexStr to Data.vi"("HEX String"=w379) -> ()  [unwired: 7 in, 2 out]
        n119 = disable-structure shown="Disabled" {
          disable-tunnel: [w384 "API2 Response"] -> w378
          frame Disabled {
            # "pack variant to hexstr \nif complex response is needed."
            # "complex Response"
            n120 = call <userlib>:"CSM - Convert Data to HexStr.vi"() -> ("HEX String (0-9,A-F)"=w384:string)  [unwired: 9 in]
          }
          frame Enabled {
          }
        }
      }
      frame "---------- DoSth ----------" {
        # "#CSM \"Category Seperator\"\nDo not put any code in this frame."
        n121 = call <vilib>:"Add State(s) to Queue__JKI_lib_State_Machine.vi"("State(s) in (\"\")"=w390) -> ("States Out"=w389:string)  [unwired: 14 in]
      }
      frame "DoSth: DoA" {
        # "#CSM \"Internal State\"\nThis category is used for holding internal states"
        n122 = call <vilib>:"Add State(s) to Queue__JKI_lib_State_Machine.vi"("State(s) in (\"\")"=w396) -> ("States Out"=w395:string)  [unwired: 14 in]
      }
      frame "DoSth: DoB" {
        # "#CSM \"Internal State\"\nThis category is used for holding internal states"
        n123 = call <vilib>:"Add State(s) to Queue__JKI_lib_State_Machine.vi"("State(s) in (\"\")"=w402) -> ("States Out"=w401:string)  [unwired: 14 in]
      }
    }
  }
